vi "Put CEID Data.vi"(8 "error in":errorcluster, 10 "CEID Data":T1, 11 "CEID":u32) -> (0 "error out":errorcluster, 3 "Find?":bool)   [LabVIEW 2020, in "SECS Communication.lvlib" / "SECS Data Class.lvclass"]
uses:
  SECS Data Class.lvclass
  CEID Data.ctl
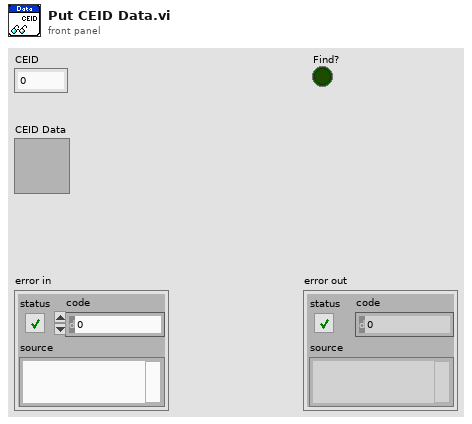
[diagram p1: front panel]
types:
  T1 = typedef "SECS Communication.lvlib/SECS Data Class.lvclass/CEID Data.ctl" = cluster{"Enable":bool, "CEID":u32, "Name":string, "Description":string, "RPTID":u32[], "Dynamic":bool}
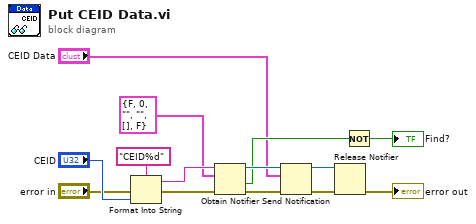
[diagram p0: block diagram]
diagram:
  n1 = Format Into String(format string="CEID%d", error in="error in", "CEID") -> (resulting string=w8:string, error out=w9:errorcluster)  [unwired: 1 in]
  n2 = Obtain Notifier(name (unnamed)=w8, notification data type=T1 {"Enable"=FALSE, "CEID"=0, "Name"="", "Description"="", "RPTID"=[], "Dynamic"=FALSE} ("CEID Data"), error in (no error)=w9) -> (notifier out=w14:refnum<notifier>, created new?=w4:bool, error out=w13:errorcluster)  [unwired: 1 in]
  n3 = Send Notification(notification="CEID Data", notifier=w14, error in (no error)=w13) -> (notifier out=w12:refnum<notifier>, error out=w11:errorcluster)
  n4 = Release Notifier(notifier=w12, error in (no error)=w11) -> (error out=→"error out":errorcluster)  [unwired: 1 in, 2 out]
  n5 = Not(x=w4) -> (.not. x?=→"Find?":bool)
